vi "SPI_Read.vi"(8 "error in (no error)":errorcluster, 9 "Read Size":u8=1, 10 "Device Register":T4 items=["WHOAMI"=0, "HW_REV"=1, "FW_VER_MAJOR"=2, "FW_VER_MINOR"=3, "UPDATE_RATE_HZ"=4, "ACCEL_FSR_G"=5, "GYRO_FSR_DPS"=6, "OP_STATUS"=8, "CAL_STATUS"=9, "SELFTEST_STATUS"=10, "CAPABILITY_FLAGS_L"=11, "CAPABILITY_FLAGS_H"=12, "SENSOR_STATUS"=16, "TIMESTAMP"=18, "YAW"=22, "ROLL"=24, "PITCH"=26, "HEADING"=28, "FUSED_HEADING"=30, "ALTITUDE_I"=32, "ALTITUDE_D"=34, "LINERA_ACC_X"=36, "LINERA_ACC_Y"=38, "LINERA_ACC_Z"=40, "QUAT_W"=42, "QUAT_X"=44, "QUAT_Y"=46, "QUAT_Z"=48, "MPU_TEMP_C"=50, "GYRO_X"=52, "GYRO_Y"=54, "GYRO_Z"=56, "ACC_X"=58, "ACC_Y"=60, "ACC_Z"=62, "MAG_X"=64, "MAG_Y"=66, "MAG_Z"=68, "PRESSURE_I"=70, "PRESSURE_D"=72, "PRESSURE_TEMP"=74, "YAW_OFFSET"=76, "QUAT_OFFSET_W"=78, "QUAT_OFFSET_X"=80, "QUAT_OFFSET_Y"=82, "QUAT_OFFSET_Z"=84, "INTEGRATION_CONTROL"=86, "VELOCITY_X"=88, "VELOCITY_Y"=92, "VELOCITY_Z"=96, "DISPLACMENT_X"=100, "DISPLACMENT_Y"=104, "DISPLACEMENT_Z"=108], 11 "SPIDevRef":T1) -> (0 "error out":errorcluster, 1 "navX Data":u8[](array[numeric]), 2 "Valid?":bool, 3 "SPIDevRef":T1={"DevStatus"={"status"=FALSE, "code"=0, "source"=""}, "Handle"=0, "Controller"=enum."Controller 1", "SPI Bus"=enum."Invalid"})   [LabVIEW 2014, in "navX Library v1 (deprecated).lvlib"]
uses:
  navX Library v1 (deprecated).lvlib
  COMMON/TypeDefs/Value TypeDefs/navX Device Registers.ctl
  <vilib>/Rock Robotics/WPI/SPI/WPI_SPIDevRef.ctl
  <vilib>/Rock Robotics/SystemInterfaces/Typedef/FPGA_TypedefDigitalModule.ctl
  <vilib>/Rock Robotics/SystemInterfaces/spilib/spi_bus.ctl
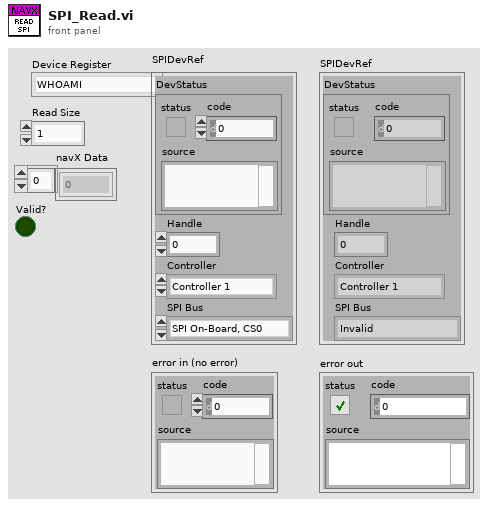
[diagram p1: front panel]
types:
  T1 = typedef "WPI_SPIDevRef.ctl" = cluster{"DevStatus":errorcluster, "Handle":i32, "Controller":T2, "SPI Bus":T3}
  T2 = typedef "FPGA_TypedefDigitalModule.ctl" = enum16{"Controller 1"}
  T3 = typedef "spi_bus.ctl" = enum16{"SPI On-Board, CS0", "SPI On-Board, CS1", "SPI On-Board, CS2", "SPI On-Board, CS3", "SPI MXP", "Invalid"}
  T4 = typedef "navX Library v1 (deprecated).lvlib/navX Device Registers.ctl" = u8
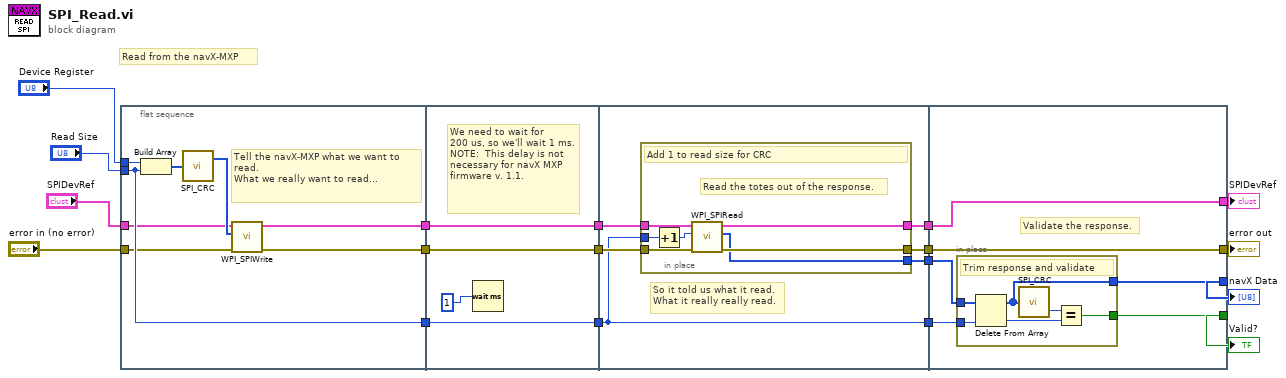
[diagram p0: block diagram]
diagram:
  # "Read from the navX-MXP"
  n1 = flat-sequence {
    tunnel: "Device Register" -> [w24]
    tunnel: "Read Size" -> [w21]
    tunnel: [w23] -> w16
    tunnel: [w22] -> w14
    tunnel: [w21] -> w6
    tunnel: "SPIDevRef" -> [w20]
    tunnel: "error in (no error)" -> [w19]
    tunnel: [w30] -> w17
    tunnel: w16 -> [w30]
    tunnel: [w29] -> w15
    tunnel: w14 -> [w29]
    tunnel: [w28] -> w7
    tunnel: w6 -> [w28]
    tunnel: w17 -> [w33]
    tunnel: w15 -> [w32]
    tunnel: [w36] -> w13
    tunnel: [w35] -> w12
    tunnel: [w34] -> w11
    tunnel: w7 -> [w31]
    tunnel: [w31] -> w5
    tunnel: [w48] -> w1
    tunnel: [w49] -> w2
    tunnel: w13 -> [w49]
    tunnel: w12 -> [w47]
    tunnel: w11 -> [w48]
    tunnel: [w46] -> w10
    tunnel: [w45] -> w9
    tunnel: w5 -> [w44]
    frame #0 {
      # "Tell the navX-MXP what we want to read.\nWhat we really want to read..."
      n2 = Build Array(w24, w21) -> (w26:T4[])
      n3 = call "SPI_CRC.vi"("Message"=w26) -> ("Message with CRC"=w25:u8[])  [unwired: 1 out]
      n4 = call <vilib>:"WPI_SPIWrite.vi"("error in (no error)"=w19, "Data To Send"=w25, "SPIDevRef"=w20) -> ("error out"=w22:errorcluster, "SPIDevRef"=w23:T1)  [unwired: 6 in, 1 out]
    }
    frame #1 {
      # "We need to wait for\n200 us, so we'll wait 1 ms.\nNOTE:  This delay is not necessary for navX MXP\nfirmware v. 1.1."
      n5 = Wait (ms)(milliseconds to wait=1) -> ()  [unwired: 1 out]
    }
    frame #2 {
      # "So it told us what it read.\nWhat it really really read."
      n6 = in-place {
        in-place-border: w32 -> [w43]
        in-place-border: w33 -> [w42]
        in-place-border: [w41] -> w36
        in-place-border: [w40] -> w34
        in-place-border: [w38] -> w35
        in-place-border: w31 -> [w37]
        # "Read the totes out of the response."
        # "Add 1 to read size for CRC"
        n7 = Increment(x=w37) -> (x+1=w39:u8)
        n8 = call <vilib>:"WPI_SPIRead.vi"("error in (no error)"=w43, "Num to Read"=w39, "SPIDevRef"=w42) -> ("error out"=w40:errorcluster, "Received Data"=w38:u8[], "SPIDevRef"=w41:T1)  [unwired: 6 in]
      }
    }
    frame #3 {
      # "Validate the response."
      n9 = in-place {
        in-place-border: [w54] -> w45
        in-place-border: w47 -> [w53]
        in-place-border: w44 -> [w52]
        in-place-border: [w50] -> w46
        # "Trim response and validate"
        n10 = Delete From Array(array=w53, index=w52) -> (deleted portion=w51:u8, array with subset deleted=w50:u8[])  [unwired: 1 in]
        n11 = call "SPI_CRC.vi"("Message"=w50) -> ("CRC"=w55:u8)  [unwired: 1 out]
        n12 = Equal?(x=w55, y=w51) -> (x = y?=w54:bool)
      }
    }
  }
  "navX Data" <- w10
  "Valid?" <- w9
  "SPIDevRef" <- w2
  "error out" <- w1
